vi "RTS Macro Defrost Peaks.vi"(7 "p":dbl=20.0 format="%#_13g", 8 "Error In":errorcluster, 11 "Time":dbl[](array[numeric])) -> (0 "Error Out":errorcluster, 2 "Number of Defrost Peaks":i32, 3 "Defrost Peaks":T1(graph))   [LabVIEW 2016]
uses:
  <vilib>/gmath/statdist.llb/st_Percentiles (scalar).vi
  <vilib>/Analysis/NI_AALPro.lvlib
  <vilib>/gmath/NI_Gmath.lvlib
panel:
  out "Array":i32[](array[numeric])
  out "Waveform Chart":dbl[](graph)
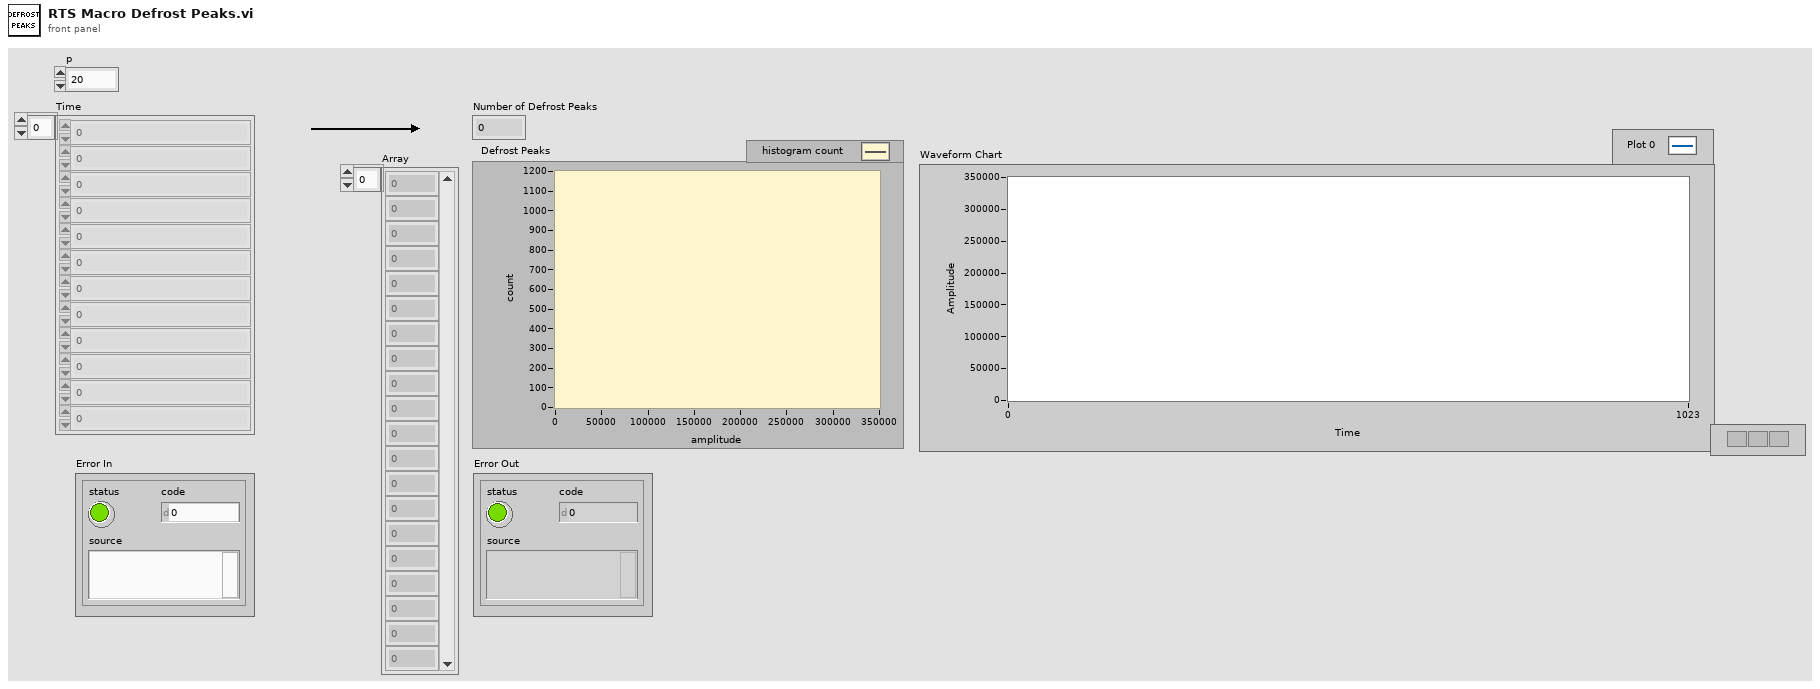
[diagram p1: front panel]
types:
  T1 = cluster{"X Values":dbl[], "Histogram: h(x)":i32[]}
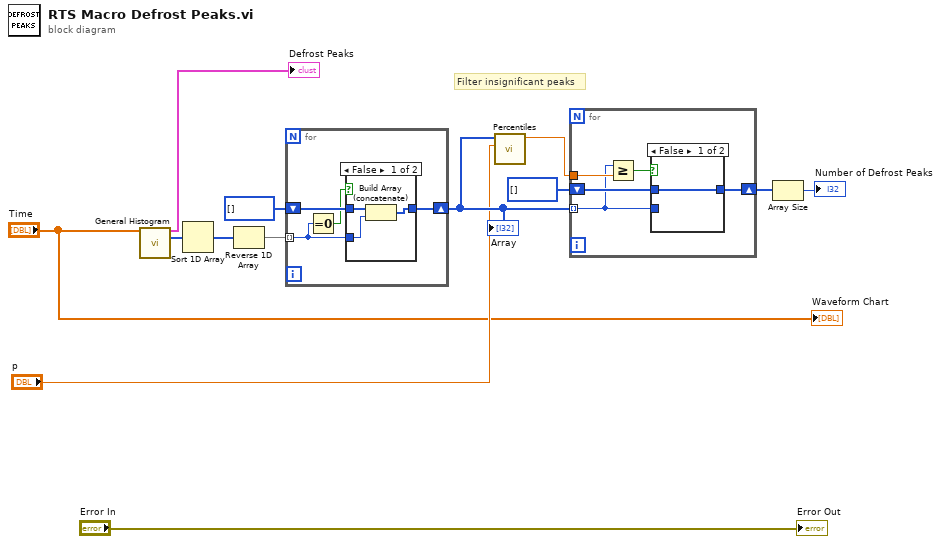
[diagram p0: block diagram]
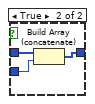
[diagram p2: hidden frame]
diagram:
  # "Filter insignificant peaks"
  n1 = call <vilib>:"General Histogram.vi"("X"="Time") -> ("Histogram Graph"=→"Defrost Peaks":T1, "Histogram"=w4:i32[])  [unwired: 10 in, 3 out]
  n2 = Sort 1D Array(array=w4) -> (sorted array=w5:i32[])
  n3 = Reverse 1D Array(array=w5) -> (reversed array=w8:i32[])
  n4 = for {
    tunnel: w8 -> [w14] mode=indexing
    shift-right: [w16] -> w9
    shift-left: i32[] [] -> [w17]
    n5 = Equal To 0?(x=w14) -> (x = 0?=w15:bool)
    n6 = case shown="False" w15 {
      tunnel: w17 -> [w20 w21]
      tunnel: [w19 w21] -> w16
      tunnel: w14 -> [w18 _]
      frame False {
        n7 = Build Array (concatenate)(w20, w18) -> (w19:i32[])
      }
      frame True {
      }
    }
  }
  "Array" <- w9
  n8 = call-poly <vilib>:"Percentiles.vi"("p"="p", "x array"=w9) -> ("percentile"=w11:dbl)  [unwired: 8 in, 1 out]
  n9 = for {
    tunnel: w9 -> [w23] mode=indexing
    tunnel: w11 -> [w26]
    shift-right: [w22] -> w12
    shift-left: i32[] [] -> [w24]
    n10 = Greater Or Equal?(x=w23, y=w26) -> (x >= y?=w25:bool)
    n11 = case shown="False" w25 {
      tunnel: w24 -> [w27 w30]
      tunnel: [w27 w29] -> w22
      tunnel: w23 -> [_ w28]
      frame False {
      }
      frame True {
        n12 = Build Array (concatenate)(w30, w28) -> (w29:i32[])
      }
    }
  }
  n13 = Array Size(array=w12) -> (size(s)=→"Number of Defrost Peaks":i32)
  "Error Out" <- "Error In"
  "Waveform Chart" <- "Time"
